vi "Read Compile Process Hook.vi"(8 "Error In":errorcluster, 11 "Context In":refnum<class "Compiler.lvclass">) -> (0 "Error Out":errorcluster, 2 "Compile Process":refnum<class "Process.lvclass">, 3 "Context Out":refnum<class "Compiler.lvclass">)   [LabVIEW 2018, in "Toolkit.lvlib" / "Compiler.lvclass"]
uses:
  Compiler.lvclass
  Hooks/Compile/Process/Process.lvclass
  Compiler.lvclass/Compiler.ctl
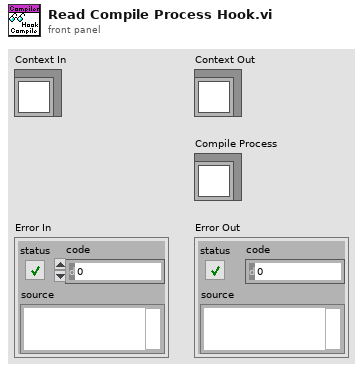
[diagram p1: front panel]
types:
  T1 = typedef "Toolkit.lvlib/Hooks.ctl" = cluster{"Compile":cluster{"Process":refnum<class "Process.lvclass">}, "Render":cluster{"Comment":refnum<class "Comment.lvclass">, "Delimiter":refnum<class "Delimiter.lvclass">, "Node":refnum<class "Node.lvclass">, "Partial":refnum<class "Partial.lvclass">, "Process":refnum<class "Process.lvclass">, "Section":refnum<class "Section.lvclass">, "Text":refnum<class "Text.lvclass">, "Variable":refnum<class "Variable.lvclass">}}
  T2 = cluster{"Process":refnum<class "Process.lvclass">}
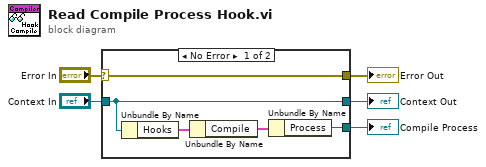
[diagram p0: block diagram]
diagram:
  n1 = case shown="No Error" "Error In" {
    selector: "Error In" -> [w10 w12]
    tunnel: "Context In" -> [w9 w11]
    tunnel: [w10 w12] -> w3
    tunnel: [w9 w11] -> w2
    tunnel: [w6 _] -> w1
    frame No Error {
      n2 = Unbundle By Name(w9) -> ("Hooks"=w8:T1)
      n3 = Unbundle By Name(w8) -> ("Compile"=w7:T2)
      n4 = Unbundle By Name(w7) -> ("Process"=w6:refnum<class "Process.lvclass">)
    }
    frame Error {
    }
  }
  "Error Out" <- w3
  "Context Out" <- w2
  "Compile Process" <- w1
